vi "Get Refs.vi"(8 "error in":errorcluster, 10 "Target Selection":string, 11 "Project in":refnum<vi>) -> (0 "error out":errorcluster, 3 "Project":refnum<class "Project.lvclass">)   [LabVIEW 2020, in "Panther Dashboard.lvlib" / "Project.lvclass"]
uses:
  Project.lvclass
  C:/GitClones/PantherDashboard/src/LabVIEW/Panther Dashboard/Class/LabVIEWItem/LabVIEWItem.lvclass
  LabVIEWItem/Item Type--enum.ctl
  LabVIEWItem/LabVIEWItem.lvclass/LabVIEWItem.ctl
  Project.lvclass/Project.ctl
  LabVIEWItem/Write Item Description.vi
  Write Project Ref.vi
  LabVIEWItem/Write Item Name.vi
  Write Target Name.vi
  Write Target Ref.vi
  Write Target App Ins Ref.vi
  Write Main App Inst Ref.vi
  LabVIEWItem/Write Item Path.vi
  LabVIEWItem/Write Item Type.vi
  Panther Dashboard/Panther Dashboard--global.vi
  LabVIEWItem/LabVIEWItem.lvclass
  Panther Dashboard/Panther Dashboard.lvlib
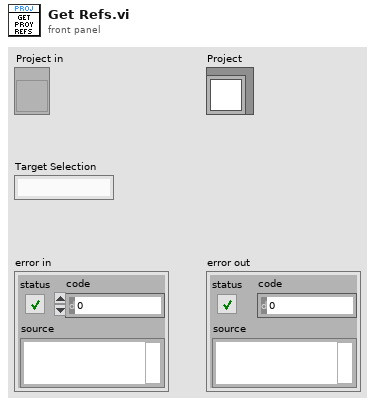
[diagram p1: front panel]
types:
  T1 = typedef "Panther Dashboard.lvlib/LabVIEWItem.lvclass/Item Type--enum.ctl" = enum16{"Requests", "Broadcasts", "Request and Wait for Reply", "Round Trip", "» Public API VIs", "» Constant VIs", "» Error VIs", "Module", "Project", "No Drag Selection"}
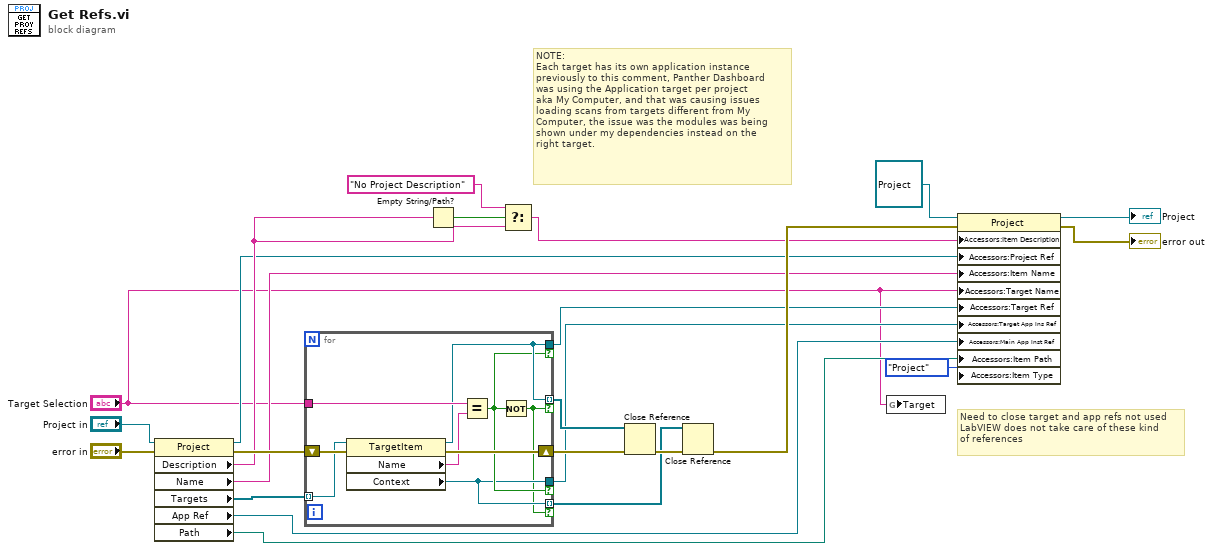
[diagram p0: block diagram]
diagram:
  # "NOTE:\nEach target has its own application instance\npreviously to this comment, Panther Dashboard\nwas using the Application target per project \naka My Computer, and that was causing issues \nloading scans from targets different from My\nComputer, the issue was the modules was being\nshown under my dependencies instead on the\nright target."
  # "Need to close target and app refs not used\nLabVIEW does not take care of these kind\nof references"
  n1 = property class="Project"(reference="Project in", error in="error in") -> (reference out=w5:refnum<vi>, error out=w22:errorcluster, "Description"=w13:string, "Name"=w10:string, "Targets"=w15:refnum<vi>[], "App Ref"=w7:refnum<vi>, "Path"=w3:path)
  n2 = for {
    tunnel: w15 -> [w31] mode=indexing
    tunnel: "Target Selection" -> [w29]
    tunnel: [w28] -> w9 if=w27
    tunnel: [w28] -> w18 mode=indexing if=w25
    shift-right: [w32] -> w21
    shift-left: w22 -> [w33]
    tunnel: [w26] -> w8 if=w27
    tunnel: [w26] -> w12 mode=indexing if=w25
    n3 = property class="TargetItem"(reference=w31, error in=w33) -> (reference out=w28:refnum<vi>, error out=w32:errorcluster, "Name"=w30:string, "Context"=w26:refnum<vi>)
    n4 = Equal?(x=w29, y=w30) -> (x = y?=w27:bool)
    n5 = Not(x=w27) -> (.not. x?=w25:bool)
  }
  n6 = Empty String/Path?(string/path=w13) -> (empty?=w16:bool)
  n7 = Select(t="No Project Description", s=w16, f=w13) -> (s? t:f=w4:string)
  n8 = Close Reference(reference=w18, error in (no error)=w21) -> (error out=w23:errorcluster)
  n9 = Close Reference(reference=w12, error in (no error)=w23) -> (error out=w20:errorcluster)
  n10 = global write "Panther Dashboard--global.vi" "Target"("Target Selection") -> ()
  n11 = property class="Project"(reference=refnum<class "Project.lvclass"> refnum ("Project.lvclass"), error in=w20, "Accessors:Item Description"=w4, "Accessors:Project Ref"=w5, "Accessors:Item Name"=w10, "Accessors:Target Name"="Target Selection", "Accessors:Target Ref"=w9, "Accessors:Target App Ins Ref"=w8, "Accessors:Main App Inst Ref"=w7, "Accessors:Item Path"=w3, "Accessors:Item Type"=Item_Type--enum."Project" ("Item Type")) -> (reference out=→"Project":refnum<class "Project.lvclass">, error out=→"error out":errorcluster)
